vi "Logging Message Loop.vi"(8 "error in (no error)":cluster{"状态":bool, "代码":i32, "源":string} caption="错误输入（无错误）", 10 "数据队列":refnum<queue>, 11 "消息队列":T1) -> (0 "error out":cluster{"状态":bool, "代码":i32, "源":string} caption="错误输出")   [LabVIEW 2012, in "Logging.lvlib"]
doc: "消息循环子VI负责处理与记录数据相关的消息。"
uses:
  Logging.lvlib
  support/Message Queue/All Message Queues.ctl
  support/Message Queue/Message Cluster.ctl
  Logging Configuration.ctl
  support/Message Queue/Message Queue.lvlib
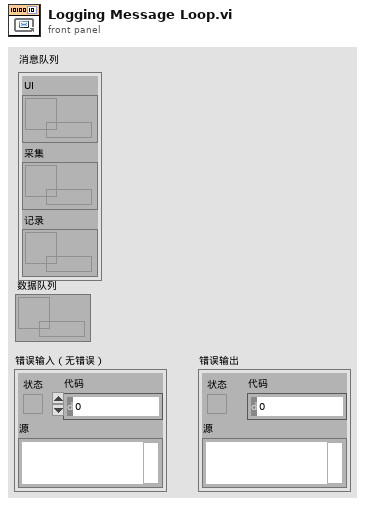
[diagram p1: front panel]
types:
  T1 = typedef "Message Queue.lvlib/All Message Queues.ctl" = cluster{"UI":refnum<queue>, "采集":refnum<queue>, "记录":refnum<queue>}
  T2 = typedef "Logging.lvlib/Logging Configuration.ctl" = cluster{"记录文件基路径":path, "TDMS文件引用":refnum<k34>}
  T3 = enum16{"open", "open or create", "create or replace", "create", "open (read-only)"}
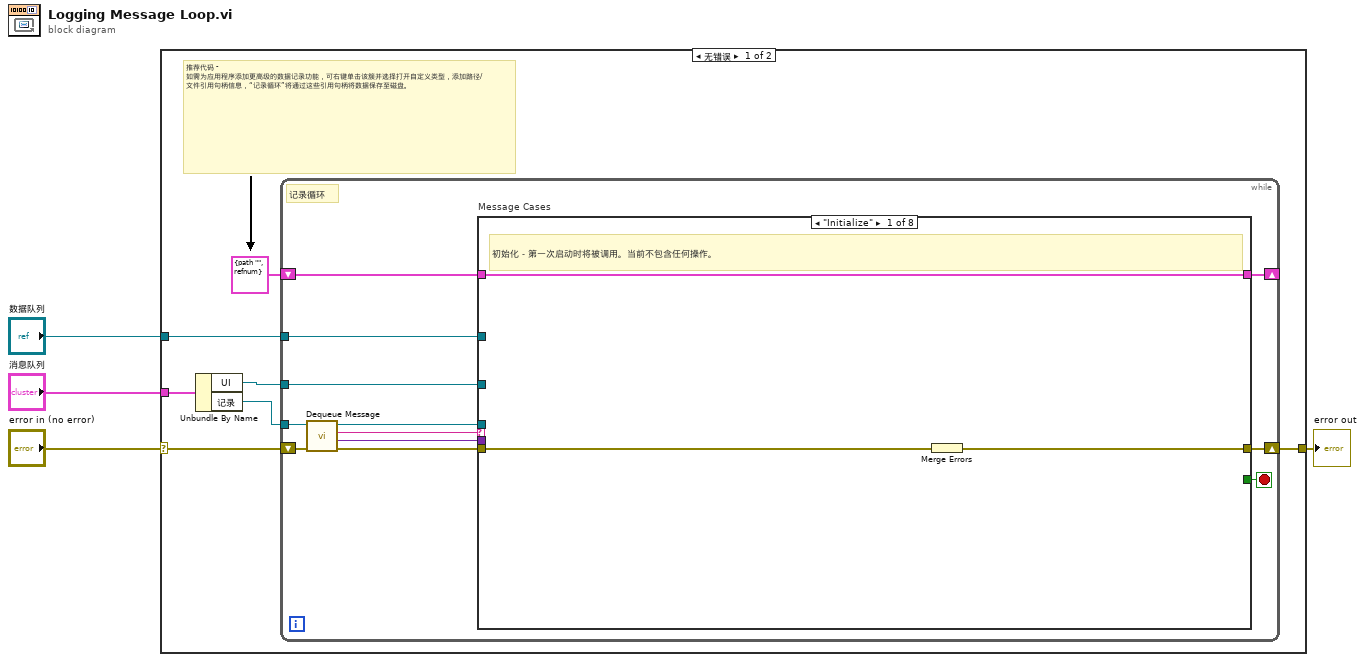
[diagram p0: block diagram]
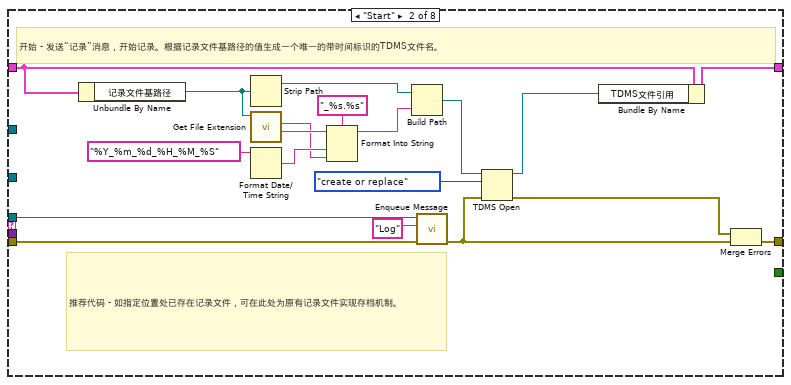
[diagram p2: hidden frame]
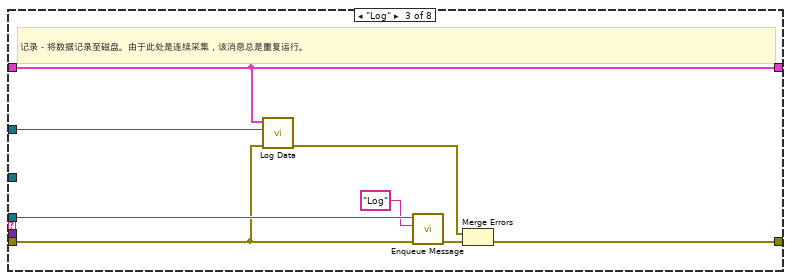
[diagram p3: hidden frame]
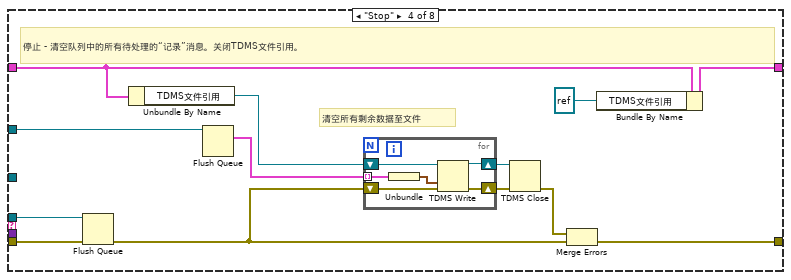
[diagram p4: hidden frame]
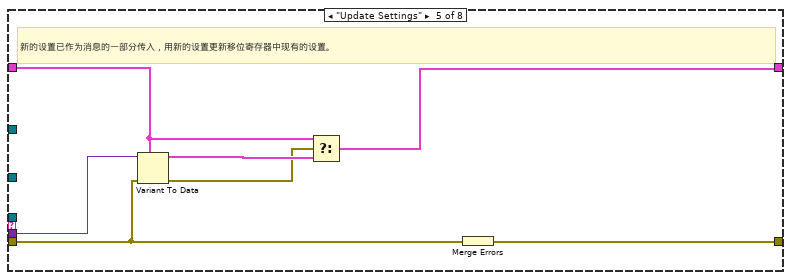
[diagram p5: hidden frame]
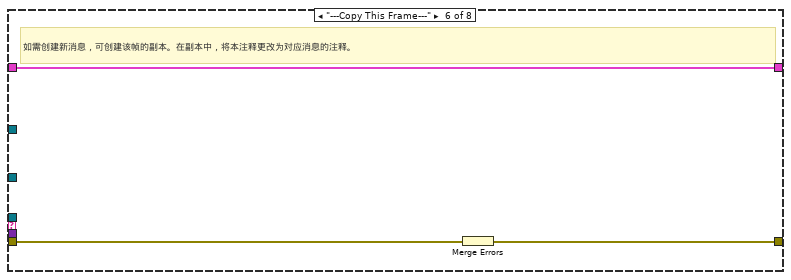
[diagram p6: hidden frame]
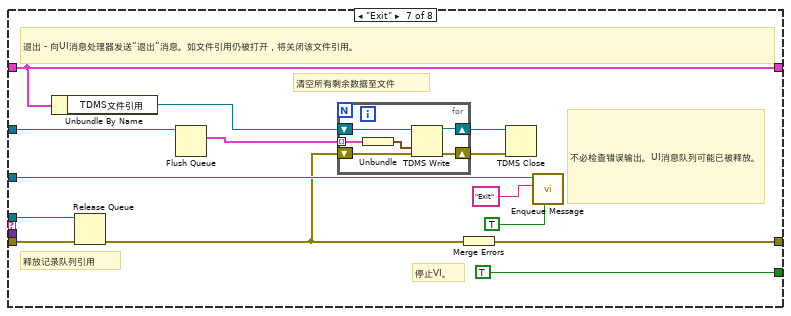
[diagram p7: hidden frame]
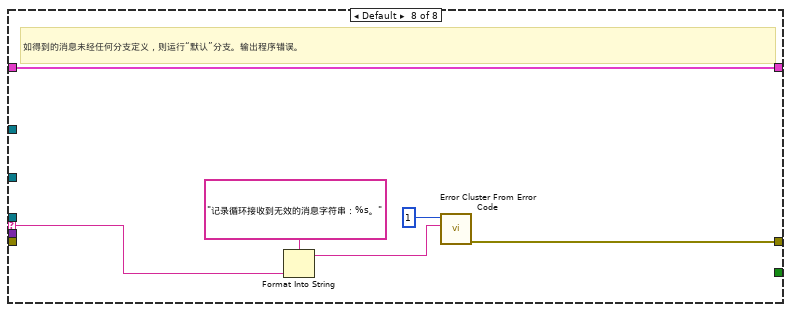
[diagram p8: hidden frame]
diagram:
  n1 = case shown="无错误" "error in (no error)" {
    selector: "error in (no error)" -> [w7 w109]
    tunnel: "消息队列" -> [w11 _]
    tunnel: [w9 w109] -> w3
    tunnel: "数据队列" -> [w6 _]
    frame No Error {
      # "推荐代码 - 如需为应用程序添加更高级的数据记录功能，可右键单击该簇并选择打开自定义类型，添加路径/文件引用句柄信息，“记录循环”将通过这些引用句柄将数据保存至磁盘。"
      n2 = Unbundle By Name(w11) -> ("UI"=w5:refnum<queue>, "记录"=w10:refnum<queue>)
      n3 = while {
        tunnel: w10 -> [w14]
        shift-right: [w22] -> _
        shift-left: T2 {"记录文件基路径"=path "", "TDMS文件引用"=refnum} ("Logging Configuration") -> [w23]
        shift-right: [w20] -> w9
        shift-left: w7 -> [w19]
        tunnel: w5 -> [w13]
        tunnel: w6 -> [w12]
        stop <- w21 stop-if-true
        # "记录循环"
        n4 = call "Dequeue Message.vi"("error in (no error)"=w19, "消息队列"=w14) -> ("error out"=w18:cluster{"状态":bool, "代码":i32, "源":string}, "消息数据"=w16:variant, "消息"=w17:string, "消息队列副本"=w15:refnum<queue>)  [unwired: 6 in]
        n5 = case "Message Cases" shown="\"Initialize\"" w17 {
          selector: w17 -> [_ _ _ _ _ _ _ w106]
          tunnel: w15 -> [_ w44 w51 w64 _ _ w90 _]
          tunnel: w18 -> [w24 w42 w48 w65 w73 w82 w93 _]
          tunnel: [w26 w45 w53 w66 w79 w80 w95 w104] -> w20
          tunnel: w23 -> [w25 w29 w46 w62 w77 w81 w89 w108]
          tunnel: [w25 w28 w46 w61 w74 w81 w89 w108] -> w22
          tunnel: [_ _ _ _ _ _ TRUE _] -> w21
          tunnel: w16 -> [_ _ _ _ w78 _ _ _]
          tunnel: w13 -> [_ _ _ _ _ _ w94 _]
          tunnel: w12 -> [_ _ w50 w59 _ _ w87 _]
          frame "Initialize" {
            # "初始化－第一次启动时将被调用。当前不包含任何操作。"
            n6 = Merge Errors(w24) -> (w26:errorcluster)
          }
          frame "Start" {
            # "开始 - 发送“记录”消息，开始记录。根据记录文件基路径的值生成一个唯一的带时间标识的TDMS文件名。"
            # "推荐代码 - 如指定位置处已存在记录文件，可在此处为原有记录文件实现存档机制。"
            n7 = Unbundle By Name(w29) -> ("记录文件基路径"=w41:path)
            n8 = Strip Path(path=w41) -> (stripped path=w38:path)  [unwired: 1 out]
            n9 = call <vilib>:"Get File Extension.vi"("file"=w41) -> ("filename without extension"=w39:string, "lowercase file extension"=w35:string)  [unwired: 7 in, 2 out]
            n10 = Format Date/Time String(time format string (%c)="%Y_%m_%d_%H_%M_%S") -> (date/time string=w36:string)  [unwired: 2 in]
            n11 = Format Into String(format string="_%s.%s", initial string=w39, w36, w35) -> (resulting string=w34:string)  [unwired: 1 in, 1 out]
            n12 = Build Path(base path=w38, name or relative path=w34) -> (appended path=w33:path)
            n13 = call "Enqueue Message.vi"("error in (no error)"=w42, "消息"="Log" ("Message"), "消息队列"=w44) -> ("error out"=w31:cluster{"状态":bool, "代码":i32, "源":string})  [unwired: 7 in, 1 out]
            n14 = TDMS Open(8:w31, 10:T3."create or replace" ("operation (0:open)"), 11:w33) -> (0:w32:errorcluster, 3:w27:refnum<k34>)  [unwired: 3 in]
            n15 = Bundle By Name(cluster=w29, "TDMS文件引用"=w27) -> (w28:T2)
            n16 = Merge Errors(w32, w31) -> (w45:errorcluster)
          }
          frame "Log" {
            # "记录－将数据记录至磁盘。由于此处是连续采集，该消息总是重复运行。"
            n17 = call "Log Data.vi"("error in (no error)"=w48, "数据队列"=w50, "记录配置"=w46) -> ("error out"=w49:cluster{"状态":bool, "代码":i32, "源":string})  [unwired: 8 in]
            n18 = call "Enqueue Message.vi"("error in (no error)"=w48, "消息"="Log" ("Message"), "消息队列"=w51) -> ("error out"=w52:cluster{"状态":bool, "代码":i32, "源":string})  [unwired: 7 in, 1 out]
            n19 = Merge Errors(w49, w52) -> (w53:errorcluster)
          }
          frame "Stop" {
            # "清空所有剩余数据至文件"
            # "停止 - 清空队列中的所有待处理的“记录”消息。关闭TDMS文件引用。"
            n20 = Flush Queue(queue=w64, error in (no error)=w65) -> (error out=w55:errorcluster)  [unwired: 2 out]
            n21 = Unbundle By Name(w62) -> ("TDMS文件引用"=w58:refnum<k34>)
            n22 = Flush Queue(queue=w59) -> (remaining elements=w54:cluster{"Array":waveform(dbl)[]}[])  [unwired: 1 in, 2 out]
            n23 = for {
              shift-right: [w69] -> w57
              shift-left: w58 -> [w70]
              shift-right: [w71] -> w56
              shift-left: w55 -> [w72]
              tunnel: w54 -> [w68] mode=indexing
              n24 = Unbundle(w68) -> ("Array"=w67:waveform(dbl)[])
              n25 = TDMS Write(0:w70, 9:w67, 11:w72) -> (4:w69:refnum<k34>, 15:w71:errorcluster)  [unwired: 3 in, 2 out]
            }
            n26 = TDMS Close(8:w56, 11:w57) -> (0:w63:errorcluster)  [unwired: 1 out]
            n27 = Merge Errors(w63, w55) -> (w66:errorcluster)
            n28 = Bundle By Name(cluster=w62, "TDMS文件引用"=refnum<k34> refnum ("TDMS File Reference")) -> (w61:T2)
          }
          frame "Update Settings" {
            # "新的设置已作为消息的一部分传入，用新的设置更新移位寄存器中现有的设置。"
            n29 = Variant To Data(error in=w73, type=w77, Variant=w78) -> (data=w76:T2, error out=w75:errorcluster)
            n30 = Select(t=w77, s=w75, f=w76) -> (s? t:f=w74:T2)
            n31 = Merge Errors(w73) -> (w79:errorcluster)
          }
          frame "---Copy This Frame---" {
            # "如需创建新消息，可创建该帧的副本。在副本中，将本注释更改为对应消息的注释。"
            n32 = Merge Errors(w82) -> (w80:errorcluster)
          }
          frame "Exit" {
            # "清空所有剩余数据至文件"
            # "释放记录队列引用"
            # "不必检查错误输出。UI消息队列可能已被释放。"
            # "停止VI。"
            # "退出 - 向UI消息处理器发送“退出”消息。如文件引用仍被打开，将关闭该文件引用。"
            n33 = Unbundle By Name(w89) -> ("TDMS文件引用"=w86:refnum<k34>)
            n34 = Release Queue(queue=w90, error in (no error)=w93) -> (error out=w85:errorcluster)  [unwired: 1 in, 2 out]
            n35 = Flush Queue(queue=w87) -> (remaining elements=w88:cluster{"Array":waveform(dbl)[]}[])  [unwired: 1 in, 2 out]
            n36 = for {
              shift-right: [w99] -> w83
              shift-left: w86 -> [w100]
              shift-right: [w101] -> w84
              shift-left: w85 -> [w102]
              tunnel: w88 -> [w98] mode=indexing
              n37 = Unbundle(w98) -> ("Array"=w97:waveform(dbl)[])
              n38 = TDMS Write(0:w100, 9:w97, 11:w102) -> (4:w99:refnum<k34>, 15:w101:errorcluster)  [unwired: 3 in, 2 out]
            }
            n39 = Merge Errors(w85) -> (w95:errorcluster)
            n40 = TDMS Close(8:w84, 11:w83) -> ()  [unwired: 2 out]
            n41 = call "Enqueue Message.vi"("优先消息？(F)"=TRUE, "消息"="Exit" ("Message"), "消息队列"=w94) -> ()  [unwired: 7 in, 2 out]
          }
          frame Default {
            # "如得到的消息未经任何分支定义，则运行“默认”分支。输出程序错误。"
            n42 = Format Into String(format string="记录循环接收到无效的消息字符串：%s。" ("Invalid Logging Message"), w106) -> (resulting string=w103:string)  [unwired: 2 in, 1 out]
            n43 = call <vilib>:"Error Cluster From Error Code.vi"("error message (\"\")"=w103, "error code (0)"=1) -> ("error out"=w104:errorcluster)  [unwired: 7 in]
          }
        }
      }
    }
    frame Error {
    }
  }
  "error out" <- w3
